vi "day 10 task 2.vi"() -> ()   [LabVIEW 2019]
panel:
  out "Part 2":bool[][](array[boolean])
  out "row (0-5)":i32
  out "during":i32[](array[numeric])
  out "sum":i32
  out "after":i32[](array[numeric])
  out "tick no.":i32
  # "1,1,4,4,-1"
  # "9-->21\n30-->19"
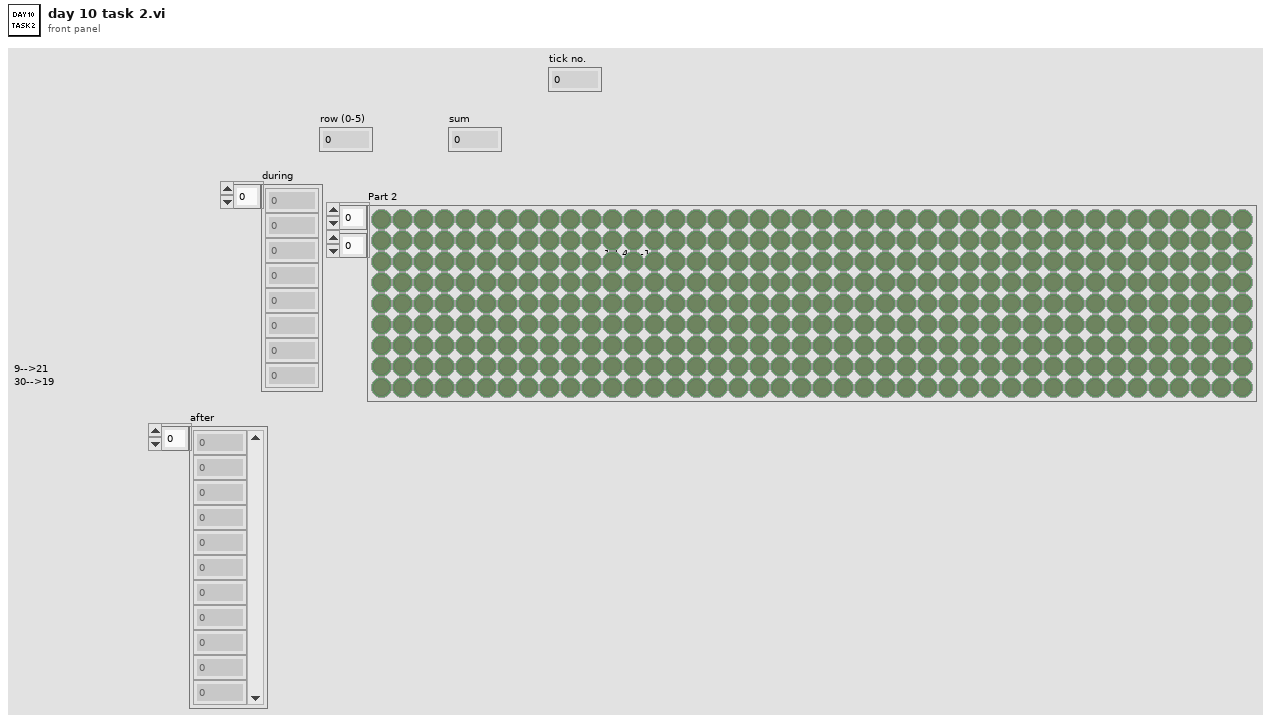
[diagram p1: front panel]
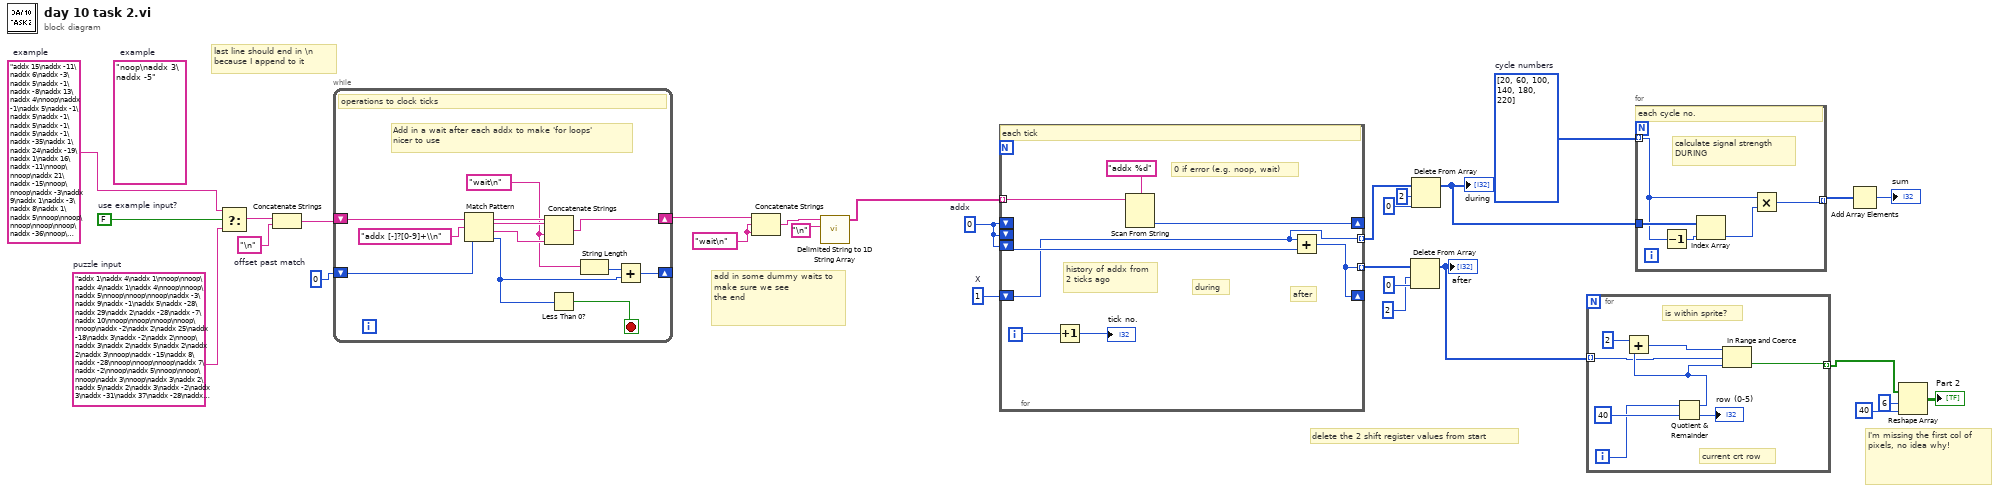
[diagram p0: block diagram]
diagram:
  w14 = i32[] [20, 60, 100, 140, 180, 220]  # cycle numbers
  w18 = "wait\n" ("regular expression")
  w20 = 1  # X
  w21 = 0  # addx
  w26 = 0  # offset past match
  w8 = "addx 15\naddx -11\naddx 6\naddx -3\naddx 5\naddx -1\naddx -8\naddx 13\naddx 4\nnoop\naddx -1\naddx 5\naddx -1\naddx 5\naddx -1\naddx 5\naddx -1\naddx 5\naddx -1\naddx -35\naddx 1\naddx 24\naddx -19\naddx 1\naddx 16\naddx -11\nnoop\nnoop\naddx 21\naddx -15\nnoop\nnoop\naddx -3\naddx 9\naddx 1\naddx -3\naddx 8\naddx 1\naddx 5\nnoop\nnoop\nnoop\nnoop\nnoop\naddx -36\nnoop\naddx 1\naddx 7\nnoop\nnoop\nnoop\naddx 2\naddx 6\nnoop\nnoop\nnoop\nnoop\nnoop\naddx 1\nnoop\nnoop\naddx 7\naddx 1\nnoop\naddx -13\naddx 13\naddx 7\nnoop\naddx 1\naddx -33\nnoop\nnoop\nnoop\naddx 2\nnoop\nnoop\nnoop\naddx 8\nnoop\naddx -1\naddx 2\naddx 1\nnoop\naddx 17\naddx -9\naddx 1\naddx 1\naddx -3\naddx 11\nnoop\nnoop\naddx 1\nnoop\naddx 1\nnoop\nnoop\naddx -13\naddx -19\naddx 1\naddx 3\naddx 26\naddx -30\naddx 12\naddx -1\naddx 3\naddx 1\nnoop\nnoop\nnoop\naddx -9\naddx 18\naddx 1\naddx 2\nnoop\nnoop\naddx 9\nnoop\nnoop\nnoop\naddx -1\naddx 2\naddx -37\naddx 1\naddx 3\nnoop\naddx 15\naddx -21\naddx 22\naddx -6\naddx 1\nnoop\naddx 2\naddx 1\nnoop\naddx -10\nnoop\nnoop\naddx 20\naddx 1\naddx 2\naddx 2\naddx -6\naddx -11\nnoop\nnoop\nnoop"  # example
  (unwired) "noop\naddx 3\naddx -5"  # example
  w28 = FALSE  # use example input?
  w29 = "addx 1\naddx 4\naddx 1\nnoop\nnoop\naddx 4\naddx 1\naddx 4\nnoop\nnoop\naddx 5\nnoop\nnoop\nnoop\naddx -3\naddx 9\naddx -1\naddx 5\naddx -28\naddx 29\naddx 2\naddx -28\naddx -7\naddx 10\nnoop\nnoop\nnoop\nnoop\nnoop\naddx -2\naddx 2\naddx 25\naddx -18\naddx 3\naddx -2\naddx 2\nnoop\naddx 3\naddx 2\naddx 5\naddx 2\naddx 2\naddx 3\nnoop\naddx -15\naddx 8\naddx -28\nnoop\nnoop\nnoop\naddx 7\naddx -2\nnoop\naddx 5\nnoop\nnoop\nnoop\naddx 3\nnoop\naddx 3\naddx 2\naddx 5\naddx 2\naddx 3\naddx -2\naddx 3\naddx -31\naddx 37\naddx -28\naddx -9\nnoop\nnoop\nnoop\naddx 37\naddx -29\naddx 4\nnoop\naddx -2\nnoop\nnoop\nnoop\naddx 7\nnoop\nnoop\nnoop\naddx 5\nnoop\nnoop\nnoop\naddx 4\naddx 2\naddx 4\naddx 2\naddx 3\naddx -2\nnoop\nnoop\naddx -34\naddx 6\nnoop\nnoop\nnoop\naddx -4\naddx 9\nnoop\naddx 5\nnoop\nnoop\naddx -2\nnoop\naddx 7\nnoop\naddx 2\naddx 15\naddx -14\naddx 5\naddx 2\naddx 2\naddx -32\naddx 33\naddx -31\naddx -2\nnoop\nnoop\naddx 1\naddx 3\naddx 2\nnoop\naddx 2\nnoop\naddx 7\nnoop\naddx 5\naddx -6\naddx 4\naddx 5\naddx 2\naddx -14\naddx 15\naddx 2\nnoop\naddx 3\naddx 4\nnoop\naddx 1\nnoop\nnoop"  # puzzle input
  # "I'm missing the first col of pixels, no idea why!"
  # "delete the 2 shift register values from start"
  # "add in some dummy waits to make sure we see \nthe end"
  # "last line should end in \\n\nbecause I append to it"
  n1 = Select(t=w8, s=w28, f=w29) -> (s? t:f=w25:string)
  n2 = Concatenate Strings(w25, "\n" ("regular expression")) -> (w23:string)
  n3 = while {
    shift-right: [w38] -> w19
    shift-left: w23 -> [w39]
    shift-right: [w34] -> _
    shift-left: w26 -> [w33]
    stop <- w40 stop-if-true
    w30 = "wait\n" ("regular expression")
    # "Add in a wait after each addx to make 'for loops'\nnicer to use"
    # "operations to clock ticks"
    n4 = Match Pattern(string=w39, regular expression="addx [-]?[0-9]+\\n", offset (0)=w33) -> (before substring=w37:string, match substring=w32:string, after substring=w36:string, offset past match=w31:i32)
    n5 = Concatenate Strings(w37, w32, w30, w36) -> (w38:string)
    n6 = Less Than 0?(x=w31) -> (x < 0?=w40:bool)
    n7 = String Length(string=w30) -> (length=w35:i32)
    n8 = Add(x=w35, y=w31) -> (x+y=w34:i32)
  }
  n9 = Concatenate Strings(w19, w18, w18) -> (w17:string)
  n10 = call <vilib>:"Delimited String to 1D String Array.vi"("delimiter"="\n", "delimited string"=w17) -> ("string array"=w22:string[])  [unwired: 9 in]
  n11 = for {
    tunnel: w22 -> [w49] mode=indexing
    shift-right: [w45] -> _
    shift-left: w21 -> [_]
    shift-left: w21 -> [_]
    shift-left: w21 -> [w44]
    shift-right: [w43] -> _
    shift-left: w20 -> [w42]
    tunnel: [w43] -> w16 mode=indexing
    tunnel: [w42] -> w11 mode=indexing
    i -> [w47]
    # "history of addx from 2 ticks ago"
    # "0 if error (e.g. noop, wait)"
    # "after"
    # "during"
    # "each tick"
    n12 = Increment(x=w47) -> (x+1=→"tick no.":i32)
    n13 = Scan From String(format string="addx %d", input string=w49) -> (output 1=w45:i32)  [unwired: 3 in, 3 out]
    n14 = Add(x=w42, y=w44) -> (x+y=w43:i32)
  }
  n15 = Delete From Array(array=w16, length=2, index=0) -> (array with subset deleted=w1:i32[])  [unwired: 1 out]
  "after" <- w1
  n16 = Delete From Array(array=w11, length=2, index=0) -> (array with subset deleted=w2:i32[])  [unwired: 1 out]
  "during" <- w2
  n17 = for {
    tunnel: w1 -> [w50] mode=indexing
    tunnel: [w52] -> w4 mode=indexing
    i -> [w54]
    # "current crt row"
    # "is within sprite?"
    n18 = Quotient & Remainder(x=w54, y=40) -> (x-y*floor(x/y)=w51:i32, floor(x/y)=→"row (0-5)":i32)
    n19 = Add(x=2, y=w51) -> (x+y=w53:i32)
    n20 = In Range and Coerce(upper limit=w53, x=w50, lower limit=w51) -> (In Range?=w52:bool)  [unwired: 1 out]
  }
  n21 = for {
    tunnel: w2 -> [w62]
    tunnel: w14 -> [w59] mode=indexing
    tunnel: [w58] -> w13 mode=indexing
    # "calculate signal strength\nDURING"
    # "each cycle no."
    n22 = Decrement(x=w59) -> (x-1=w61:i32)
    n23 = Index Array(array=w62, index=w61) -> (element=w60:i32)
    n24 = Multiply(x=w59, y=w60) -> (x*y=w58:i32)
  }
  n25 = Add Array Elements(numeric array=w13) -> (sum=→"sum":i32)
  n26 = Reshape Array(w4, 6 ("dimension size"), 40 ("dimension size")) -> (→"Part 2":bool[][])
